vi "Text_for_latex.vi"(1 "Input String":string) -> (0 "Output String":string)   [LabVIEW 2013]
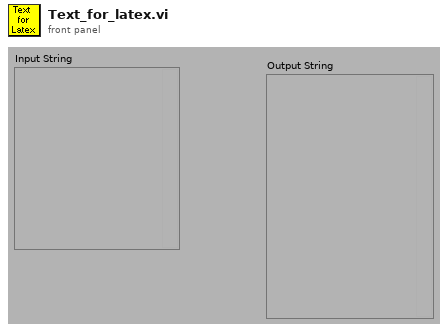
[diagram p1: front panel]
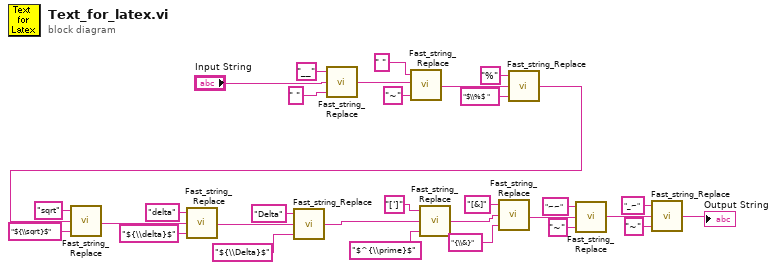
[diagram p0: block diagram]
diagram:
  n1 = call "Fast_string_Replace.vi"("Replace match with:"=" ", "Input String"="Input String", "regular expression"="__") -> ("Output String"=w5:string)  [unwired: 2 out]
  n2 = call "Fast_string_Replace.vi"("Replace match with:"="~", "Input String"=w5, "regular expression"=" ") -> ("Output String"=w16:string)  [unwired: 2 out]
  n3 = call "Fast_string_Replace.vi"("Replace match with:"="$\\%$ ", "Input String"=w16, "regular expression"="%") -> ("Output String"=w10:string)  [unwired: 2 out]
  n4 = call "Fast_string_Replace.vi"("Replace match with:"="${\\sqrt}$", "Input String"=w10, "regular expression"="sqrt") -> ("Output String"=w9:string)  [unwired: 2 out]
  n5 = call "Fast_string_Replace.vi"("Replace match with:"="${\\delta}$", "Input String"=w9, "regular expression"="delta") -> ("Output String"=w23:string)  [unwired: 2 out]
  n6 = call "Fast_string_Replace.vi"("Replace match with:"="${\\Delta}$", "Input String"=w23, "regular expression"="Delta") -> ("Output String"=w24:string)  [unwired: 2 out]
  n7 = call "Fast_string_Replace.vi"("Replace match with:"="$^{\\prime}$", "Input String"=w24, "regular expression"="[']") -> ("Output String"=w19:string)  [unwired: 2 out]
  n8 = call "Fast_string_Replace.vi"("Replace match with:"="{\\&}", "Input String"=w19, "regular expression"="[&]") -> ("Output String"=w13:string)  [unwired: 2 out]
  n9 = call "Fast_string_Replace.vi"("Replace match with:"="~", "Input String"=w13, "regular expression"="~~") -> ("Output String"=w2:string)  [unwired: 2 out]
  n10 = call "Fast_string_Replace.vi"("Replace match with:"="~", "Input String"=w2, "regular expression"="_~") -> ("Output String"=→"Output String":string)  [unwired: 2 out]
